vi "Auto_Routine_Triangle.vi"(8 "error in (no error)":errorcluster) -> (0 "error out":errorcluster)   [LabVIEW 2023]
doc: "Drives in a triangle\n\ninputs:\n--ErrorIn--\n\noutputs:\n--ErrorOut"
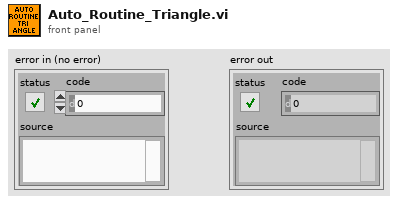
[diagram p1: front panel]
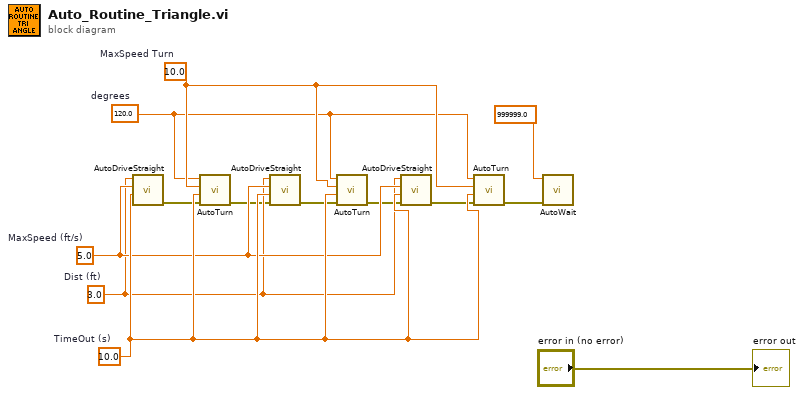
[diagram p0: block diagram]
diagram:
  w12 = 10.0  # TimeOut (s)
  w11 = 10.0  # MaxSpeed Turn
  w10 = 5.0  # MaxSpeed (ft/s)
  w9 = 120.0  # degrees
  w8 = 3.0  # Dist (ft)
  n1 = call "AutoDriveStraight.vi"("TimeOut (s)"=w12, "MaxSpeed (ft/s)"=w10, "Dist (ft)"=w8) -> ("error out"=w2:errorcluster)  [unwired: 8 in]
  n2 = call "AutoTurn.vi"("error in (no error)"=w2, "TimeOut (s)"=w12, "MaxSpeed (ft/s)"=w11, "degrees"=w9) -> ("error out"=w3:errorcluster)  [unwired: 7 in]
  n3 = call "AutoDriveStraight.vi"("error in (no error)"=w3, "TimeOut (s)"=w12, "MaxSpeed (ft/s)"=w10, "Dist (ft)"=w8) -> ("error out"=w4:errorcluster)  [unwired: 7 in]
  n4 = call "AutoTurn.vi"("error in (no error)"=w4, "TimeOut (s)"=w12, "MaxSpeed (ft/s)"=w11, "degrees"=w9) -> ("error out"=w5:errorcluster)  [unwired: 7 in]
  n5 = call "AutoDriveStraight.vi"("error in (no error)"=w5, "TimeOut (s)"=w12, "MaxSpeed (ft/s)"=w10, "Dist (ft)"=w8) -> ("error out"=w6:errorcluster)  [unwired: 7 in]
  n6 = call "AutoTurn.vi"("error in (no error)"=w6, "TimeOut (s)"=w12, "MaxSpeed (ft/s)"=w11, "degrees"=w9) -> ("error out"=w7:errorcluster)  [unwired: 7 in]
  n7 = call "AutoWait.vi"("error in (no error)"=w7, "TimeOut (s)"=999999.0) -> ()  [unwired: 9 in, 1 out]
  "error out" <- "error in (no error)"
